vi "PID_Planta.vi"() -> ()   [LabVIEW 2010]
panel:
  out "U":dbl
  in  "td (sec)":dbl
  in  "ti (sec)":dbl
  in  "kp":dbl
  out "Waveform Chart":cluster{"h":dbl, "SetPoint":dbl}(graph)
  in  "Automatico_ON/Manual_OFF":bool=TRUE
  in  "umanual":dbl(slide) scale=0.0..10.0
  in  "PID default parameters":T1={"kp"=20.0, "ti (sec)"=0.8, "td (sec)"=0.0, "N"=1.0, "tt"=10.0, "beta"=1.0}
  in  "dt":dbl=0.1
  in  "SetPoint":dbl(slide)=0.05 scale=0.0..0.2
  out "Nivel":dbl(slide)=0.1 scale=0.0..0.2
  in  "stop":bool
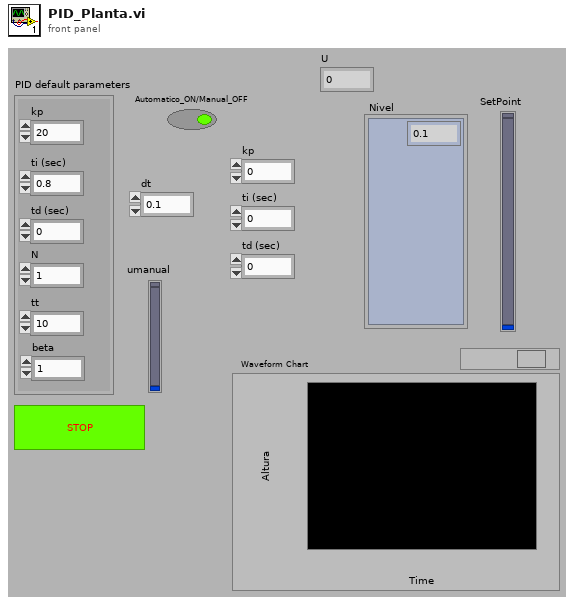
[diagram p1: front panel]
types:
  T1 = cluster{"kp":dbl, "ti (sec)":dbl, "td (sec)":dbl, "N":dbl, "tt":dbl, "beta":dbl}
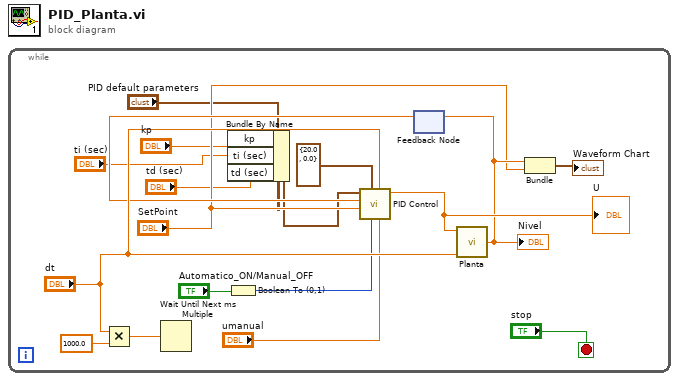
[diagram p0: block diagram]
diagram:
  n1 = while {
    stop <- "stop" stop-if-true
    n2 = Multiply(x="dt", y=1000.0) -> (x*y=w16:dbl)
    n3 = Wait Until Next ms Multiple(millisecond multiple=w16) -> ()  [unwired: 1 out]
    n4 = Bundle By Name(cluster="PID default parameters", "kp"="kp", "ti (sec)"="ti (sec)", "td (sec)"="td (sec)") -> (w4:T1)
    n5 = Boolean To (0,1)(Boolean="Automatico_ON/Manual_OFF") -> (0, 1=w9:i16)
    n6 = feedback #1() -> (w12:dbl)  [unwired: 1 in]
    n7 = call "PID Control.vi"("umanual"="umanual", "dt (sec)"="dt", "manual"=w9, "output limit"=cluster{"umax":dbl, "umin":dbl} {"umax"=20.0, "umin"=0.0}, "setpoint"="SetPoint", "process variable"=w12, "PID parameters"=w4) -> ("usat"=w11:dbl)  [unwired: 4 in]
    "U" <- w11
    n8 = call "Planta.vi"("u"=w11, "dt"="dt") -> ("h"=w8:dbl)  [unwired: 3 in]
    "Nivel" <- w8
    n9 = feedback-in #1(w8) -> ()
    n10 = Bundle("h"=w8, "SetPoint"="SetPoint") -> (→"Waveform Chart":cluster{"h":dbl, "SetPoint":dbl})  [unwired: 1 in]
  }
